vi "本地数字信号仿真.vi"() -> ()   [LabVIEW 2012]
uses:
  <vilib>/ptbypt/Frequency Domain.llb/Real FFT PtByPt.vi
  <vilib>/ptbypt/NI_PtbyPt.lvlib
  <vilib>/Analysis/NI_AALBase.lvlib
panel:
  out "Last Element Inserted 3.78MHz":dbl caption="最后插入的元素" format="%0.2f"
  out "Last Element Removed 3.78MHz":dbl caption="最后删除的元素" format="%0.2f"
  out "Last Element Inserted":dbl caption="最后插入的元素" format="%0.2f"
  out "Last Element Removed":dbl caption="最后删除的元素" format="%0.2f"
  out "Elements in Queue":i32(slide) caption="队列中的元素" scale=0.0..60000000.0 scale format="%0.0f"
  out "Waveform Chart":cluster{"Last Element Inserted":dbl, dbl}(graph) caption="波形图表"
  out "Elements in Queue 2":i32(slide) caption="队列中的元素" scale=0.0..60000000.0 scale format="%0.0f"
  out "Waveform Chart 2":cluster{"Last Element Inserted":dbl, dbl}(graph) caption="波形图表"
  in  "Queue Size":i32=60000000 caption="队列大小"
  in  "退出":bool
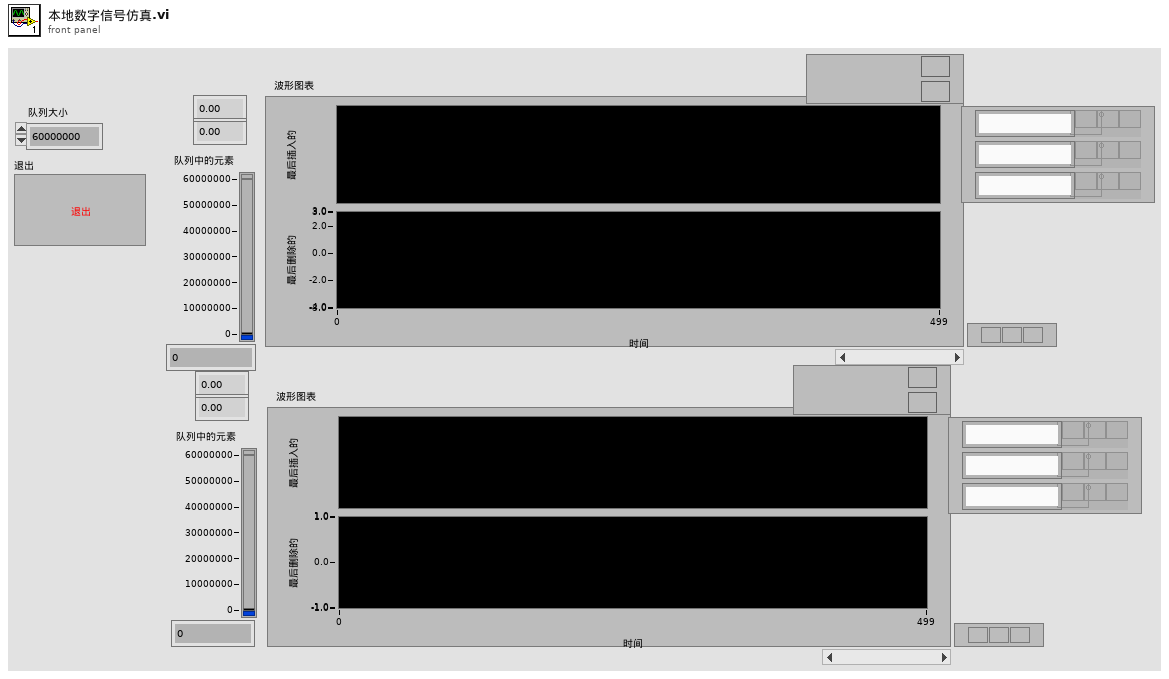
[diagram p1: front panel]
types:
  T1 = cluster{"Last Element Inserted":dbl, "Last Element Removed":dbl}
  T2 = cluster{"Last Element Inserted 3.78MHz":dbl, "Last Element Removed 3.78MHz":dbl}
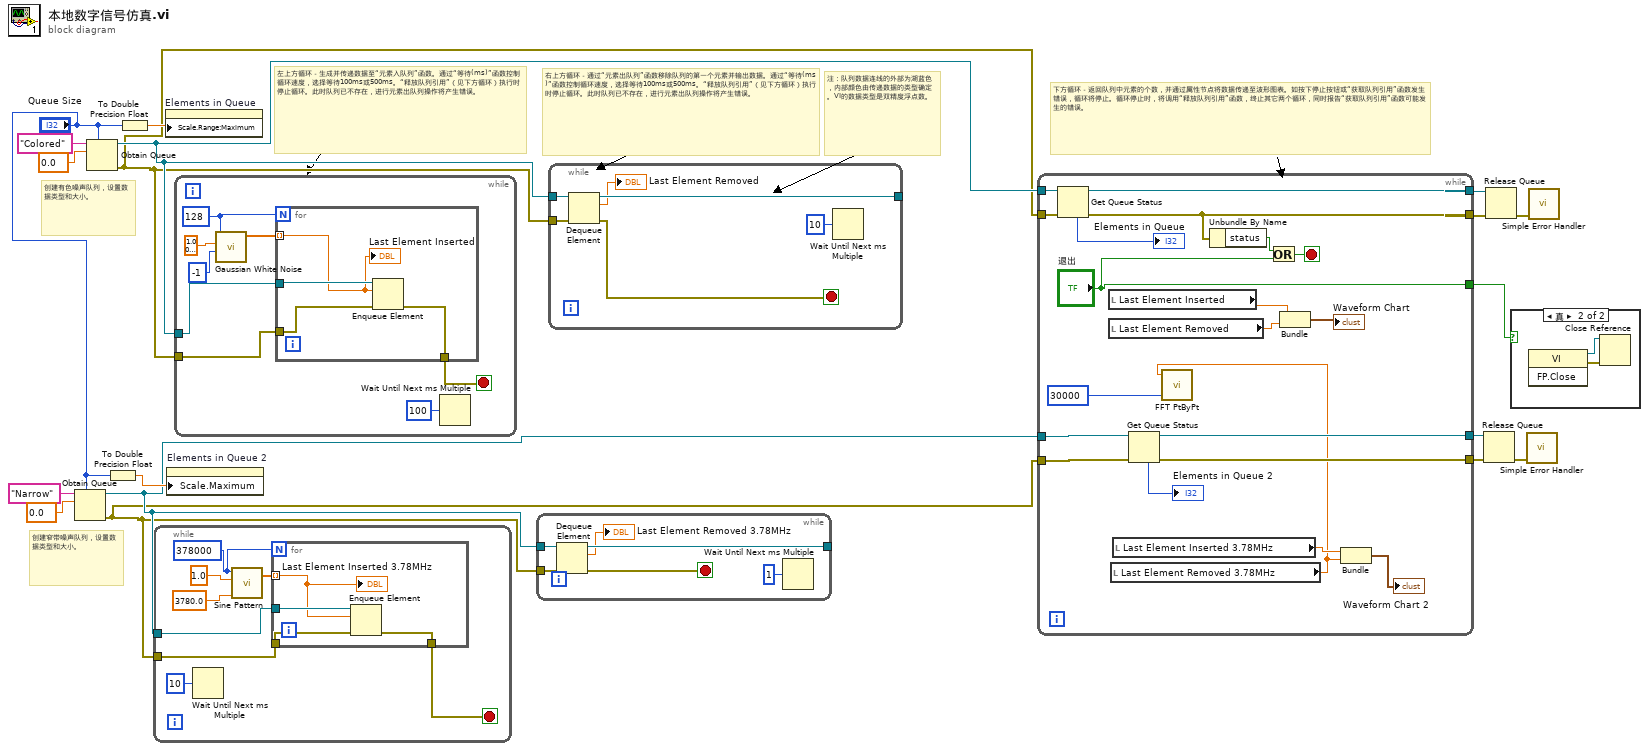
[diagram p0: block diagram]
diagram:
  # "创建窄带噪声队列，设置数据类型和大小。"
  # "右上方循环－通过“元素出队列”函数移除队列的第一个元素并输出数据。通过“等待(ms)”函数控制循环速度，选择等待100ms或500ms。“释放队列引用”（见下方循环）执行时停止循环。此时队列已不存在，进行元素出队列操作将产生错误。"
  # "注：队列数据连线的外部为湖蓝色，内部颜色由传递数据的类型确定。VI的数据类型是双精度浮点数。"
  # "下方循环－返回队列中元素的个数，并通过属性节点将数据传递至波形图表。如按下停止按钮或“获取队列引用”函数发生错误，循环将停止。循环停止时，将调用“释放队列引用”函数，终止其它两个循环，同时报告“获取队列引用”函数可能发生的错误。"
  # "左上方循环－生成并传递数据至“元素入队列”函数。通过“等待(ms)”函数控制循环速度，选择等待100ms或500ms。“释放队列引用”（见下方循环）执行时停止循环。此时队列已不存在，进行元素出队列操作将产生错误。"
  # "创建有色噪声队列，设置数据类型和大小。"
  n1 = Obtain Queue(max queue size (-1, unlimited)="Queue Size", name (unnamed)="Narrow", element data type=0.0) -> (queue out=w3:refnum<queue>, error out=w2:errorcluster)  [unwired: 2 in, 1 out]
  n2 = Obtain Queue(max queue size (-1, unlimited)="Queue Size", name (unnamed)="Colored", element data type=0.0) -> (queue out=w5:refnum<queue>, error out=w4:errorcluster)  [unwired: 2 in, 1 out]
  n3 = To Double Precision Float(number="Queue Size") -> (double precision float=w11:dbl)
  n4 = To Double Precision Float(number="Queue Size") -> (double precision float=w18:dbl)
  n5 = while {
    tunnel: w3 -> [w26]
    tunnel: w2 -> [w25]
    stop <- w19 stop-if-true
    w20 = 378000 ("samples")
    n6 = Wait Until Next ms Multiple(millisecond multiple=u32 10 ("milliseconds to wait")) -> ()  [unwired: 1 out]
    n7 = call <vilib>:"Sine Pattern.vi"("cycles"=3780.0, "amplitude"=1.0, "samples"=w20) -> ("Sinusoidal Pattern"=w21:dbl[])  [unwired: 1 in, 1 out]
    n8 = for {
      N: w20 -> [_]
      tunnel: w26 -> [w30]
      tunnel: w25 -> [w29]
      tunnel: [w28] -> w19
      tunnel: w21 -> [w27] mode=indexing
      n9 = Enqueue Element(queue=w30, element=w27, error in (no error)=w29) -> (error out=w28:errorcluster)  [unwired: 3 out]
      "Last Element Inserted 3.78MHz" <- w27
    }
  }
  n10 = property on="Elements in Queue" class="Slide (严格)"("Scale.Range:Maximum"=w18) -> ()  [unwired: 2 in, 2 out]
  n11 = property on="Elements in Queue 2" class="Slide (严格)"("Scale.Maximum"=w11) -> ()  [unwired: 2 in, 2 out]
  n12 = while {
    tunnel: w5 -> [w34]
    tunnel: w4 -> [w33]
    stop <- w35 stop-if-true
    w36 = 128 ("samples")
    n13 = call <vilib>:"Gaussian White Noise.vi"("seed"=-1, "standard deviation"=1.0000000000000002, "samples"=w36) -> ("Gaussian noise pattern"=w32:dbl[])  [unwired: 7 in, 1 out]
    n14 = for {
      N: w36 -> [_]
      tunnel: [w42] -> w35
      tunnel: w34 -> [w41]
      tunnel: w33 -> [w40]
      tunnel: w32 -> [w39] mode=indexing
      n15 = Enqueue Element(queue=w41, element=w39, error in (no error)=w40) -> (error out=w42:errorcluster)  [unwired: 3 out]
      "Last Element Inserted" <- w39
    }
    n16 = Wait Until Next ms Multiple(millisecond multiple=u32 100 ("milliseconds to wait")) -> ()  [unwired: 1 out]
  }
  n17 = while {
    tunnel: w3 -> [w48]
    tunnel: [w47] -> _
    tunnel: w2 -> [w46]
    stop <- w43 stop-if-true
    n18 = Dequeue Element(queue=w48, error in (no error)=w46) -> (queue out=w47:refnum<queue>, element=→"Last Element Removed 3.78MHz":dbl, error out=w43:errorcluster)  [unwired: 2 out]
    n19 = Wait Until Next ms Multiple(millisecond multiple=u32 1 ("milliseconds to wait")) -> ()  [unwired: 1 out]
  }
  n20 = while {
    tunnel: w5 -> [w54]
    tunnel: [w53] -> _
    tunnel: w4 -> [w52]
    stop <- w49 stop-if-true
    n21 = Dequeue Element(queue=w54, error in (no error)=w52) -> (queue out=w53:refnum<queue>, element=→"Last Element Removed":dbl, error out=w49:errorcluster)  [unwired: 2 out]
    n22 = Wait Until Next ms Multiple(millisecond multiple=u32 10 ("milliseconds to wait")) -> ()  [unwired: 1 out]
  }
  n23 = while {
    tunnel: w5 -> [w74]
    tunnel: [w67] -> w15
    tunnel: w4 -> [w70]
    tunnel: [w68] -> w14
    tunnel: w3 -> [w61]
    tunnel: w2 -> [w60]
    tunnel: [w59] -> w7
    tunnel: [w58] -> w6
    tunnel: ["退出"] -> w1
    stop <- w72 stop-if-true
    n24 = Get Queue Status(queue=w74, error in (no error)=w70) -> (queue out=w68:refnum<queue>, error out=w67:errorcluster, # elements in queue=→"Elements in Queue":i32)  [unwired: 6 out]
    n25 = local read "Last Element Inserted"() -> (w69:dbl)
    n26 = local read "Last Element Removed"() -> (w65:dbl)
    n27 = local read "Last Element Removed 3.78MHz"() -> (w56:dbl)
    n28 = local read "Last Element Inserted 3.78MHz"() -> (w63:dbl)
    n29 = Get Queue Status(queue=w61, error in (no error)=w60) -> (queue out=w59:refnum<queue>, error out=w58:errorcluster, # elements in queue=→"Elements in Queue 2":i32)  [unwired: 6 out]
    n30 = call-poly <vilib>:"FFT PtByPt.vi"("sample length"=30000, "x"=w56) -> ()  [unwired: 2 in, 2 out]
    n31 = Unbundle By Name(w67) -> ("status"=w71:bool)
    n32 = Or(x=w71, y="退出") -> (x .or. y?=w72:bool)
    n33 = Bundle("Last Element Inserted"=w69, "Last Element Removed"=w65) -> (→"Waveform Chart":T1)  [unwired: 1 out]
    n34 = Bundle("Last Element Inserted 3.78MHz"=w63, "Last Element Removed 3.78MHz"=w56) -> (→"Waveform Chart 2":T2)  [unwired: 1 out]
  }
  n35 = Release Queue(queue=w7, error in (no error)=w6) -> (error out=w8:errorcluster)  [unwired: 3 out]
  n36 = Release Queue(queue=w14, error in (no error)=w15) -> (error out=w10:errorcluster)  [unwired: 3 out]
  n37 = case shown="真" w1 {
    frame False {
    }
    frame True {
      n38 = invoke class="VI" method="FP.Close"() -> (reference out=w75:refnum<vi>, error out=w76:errorcluster)  [unwired: 3 in, 1 out]
      n39 = Close Reference(reference=w75, error in (no error)=w76) -> ()  [unwired: 1 out]
    }
  }
  n40 = call <vilib>:"Simple Error Handler.vi"("error in (no error)"=w8) -> ()  [unwired: 1 in, 8 out]
  n41 = call <vilib>:"Simple Error Handler.vi"("error in (no error)"=w10) -> ()  [unwired: 1 in, 8 out]
